vi "Track Service.vi"(0 "Room Service Monitor Model in":refnum<class "Room Service Monitor Model.lvclass">, 5 "Rooms No":string, 7 "Room Service":refnum<class "Room Service Base.lvclass">, 11 "error in (no error)":errorcluster) -> (4 "Room Service Monitor Model out":refnum<class "Room Service Monitor Model.lvclass">, 15 "error out":errorcluster)   [LabVIEW 2023, in "Room Service Monitor Model.lvlib" / "Room Service Monitor Model.lvclass"]
uses:
  Room Service Monitor Model.lvclass
  Room Service Types/Room Service Base/Room Service Base.lvclass
  Room Service Monitor Model.lvclass/Room Service Monitor Model.ctl
  <vilib>/ActorFramework/Actor/Actor.lvclass
  Room Service Monitor Model Messages/Check Staff Msg/Check Staff Msg.lvclass
  C:/Users/bhaghyaraj/Trainings/NI Actor Framework/SDLC/Model Base/Model Base/Model Base.lvclass
  C:/Program Files/National Instruments/LabVIEW 2023/vi.lib/ActorFramework/Actor/Actor.lvclass
  C:/Users/bhaghyaraj/Trainings/NI Actor Framework/SDLC/Interfaces/Model Base/Incoming Model Base Interface.lvclass
  C:/Users/bhaghyaraj/Trainings/NI Actor Framework/SDLC/Room Service Monitor Model/Room Service Monitor Model/Room Service Monitor Model.lvclass
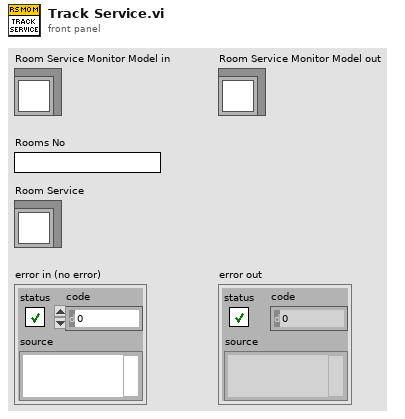
[diagram p1: front panel]
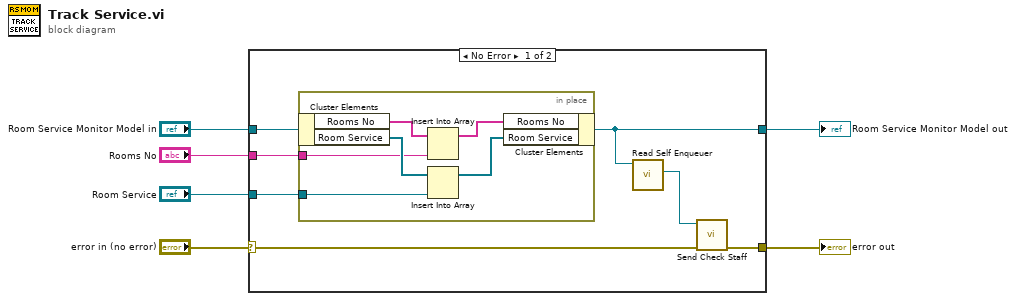
[diagram p0: block diagram]
diagram:
  n1 = case shown="No Error" "error in (no error)" {
    selector: "error in (no error)" -> [w12 w21]
    tunnel: [w8 w21] -> w5
    tunnel: [w9 w20] -> w3
    tunnel: "Room Service Monitor Model in" -> [w13 w20]
    tunnel: "Rooms No" -> [w11 _]
    tunnel: "Room Service" -> [w10 _]
    frame No Error {
      n2 = in-place {
        in-place-border: w11 -> [w15]
        in-place-border: w10 -> [w14]
        n3 = in-place-cluster #1(w13) -> ("Rooms No"=w19:string[], "Room Service"=w17:refnum<class "Room Service Base.lvclass">[])
        n4 = Insert Into Array(array=w19, new element=w15) -> (w18:string[])  [unwired: 1 in]
        n5 = Insert Into Array(array=w17, new element=w14) -> (w16:refnum<class "Room Service Base.lvclass">[])  [unwired: 1 in]
        n6 = in-place-cluster #1("Rooms No"=w18, "Room Service"=w16) -> (w9:refnum<class "Room Service Monitor Model.lvclass">)
      }
      n7 = call <vilib>:"Read Self Enqueuer.vi"("Actor"=w9) -> ("Self Enqueuer"=w7:refnum<class "Message Enqueuer.lvclass">)  [unwired: 10 in]
      n8 = call "Send Check Staff.vi"("error in (no error)"=w12, "Message Enqueuer"=w7) -> ("error out"=w8:errorcluster)  [unwired: 8 in, 1 out]
    }
    frame Error {
    }
  }
  "error out" <- w5
  "Room Service Monitor Model out" <- w3
